vi "serial_02.vi"(0 "VISA resource name":refnum<visa-resource-name>="COM5") -> ()   [LabVIEW 2010]
doc: "The Basic Serial Read and Write example performs a Serial Port Read, a Serial Port Write, or a combination of these actions. The user selects the actions (read or write) on the front panel. If both are selected, the VI will write the data first, read data, and then close the VISA session that is opened to the port. This VI will wait until the specified number of bytes is received at the port. Only the number of bytes specified will be read.\n\nINSTRUCTIONS:\n1) Select the serial resource and configuration parameters (baud rate, data bits, parity, stop bits, flow control).\n2) Select the operations to be performed. \n3) Connect the serial port to your device. If no device is available, perform a loopback test by doing one of the following. Short pins 2 and 3 on a RS-232 cable or short pin 4 to pin 8 and pin 5 to pin 9 on a RS-485/422 cable. \n4) Run the VI to see the data read. (The \"read string\" will match the \"string to write\" if a loopback test was performed.)\n\nNote: The parameters set for the serial port must match the parameters of the connected instrument or device. In this example, the bytes to read parameter specifies the number of bytes that the serial port reads. If there were more bytes at the port than the number specified in bytes to read, those bytes would not be read. Also, if you specify to read more bytes than the number of bytes actually read, you might receive a timeout error message.\n\nOn the block diagram, the Configure Serial Port VI sets the configuration parameters. The front panel displays the controls used to configure the basic parameters, such as baud rate, data bits, and parity. Constants configure the other parameters the user probably does not need set. After the VISA Configure Serial Port VI opens the VISA session and configures the port, the VI passes the VISA resource name to other VIs that perform operations on that VISA resource. The VISA Write function sends a command to the serial device and the VISA Read function returns data based on the command. The VISA Close function then closes the reference to the serial device. It is important to close the reference; otherwise communication through with that port through protocols other than VISA might not be possible."
panel:
  in  "Start":bool=TRUE
  out "Meter":dbl(knob)=668.0 scale=0.0..1024.0
  out "Waveform Chart":i32(graph)=668
  # "Stop"
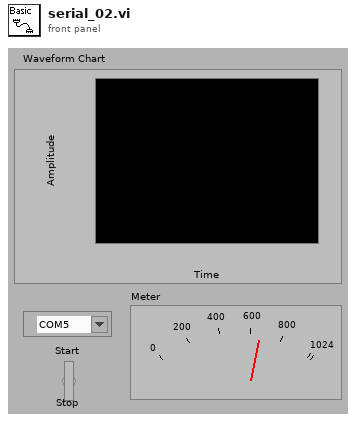
[diagram p1: front panel]
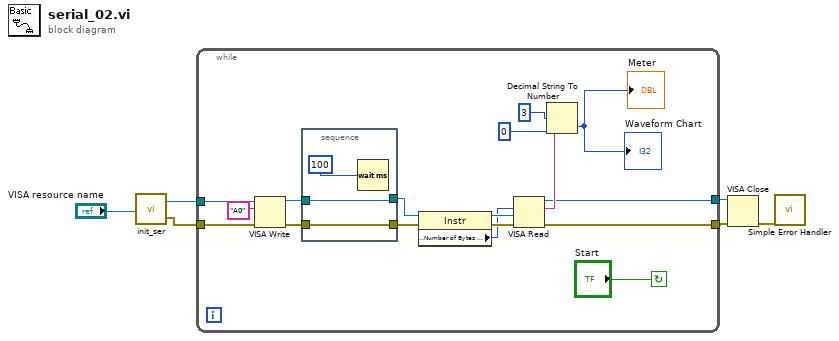
[diagram p0: block diagram]
diagram:
  n1 = call "init_ser.vi"("VISA resource name"="VISA resource name") -> ("VISA resource name out"=w4:refnum<visa-resource-name>, "error out"=w5:errorcluster)
  n2 = while {
    tunnel: w5 -> [w20]
    tunnel: w4 -> [w21]
    tunnel: [w9] -> w3
    tunnel: [w10] -> w2
    stop <- "Start" continue-if-true
    n3 = VISA Write(VISA resource name=w21, write buffer="A0" ("string to write"), error in (no error)=w20) -> (VISA resource name out=w19:refnum<visa-resource-name>, error out=w18:errorcluster)  [unwired: 1 out]
    n4 = stacked-sequence {
      tunnel: w19 -> [w25]
      tunnel: w18 -> [w24]
      tunnel: [w25] -> w8
      tunnel: [w24] -> w7
      frame #0 {
        n5 = Wait (ms)(milliseconds to wait=u32 100 ("delay before read (ms)")) -> ()  [unwired: 1 out]
      }
    }
    n6 = property class="Instr"(reference=w8, error in=w7) -> (reference out=w17:refnum<visa-resource-name>, error out=w16:errorcluster, "Serial Settings:Number of Bytes at Serial Port"=w15:u32)
    n7 = VISA Read(VISA resource name=w17, byte count=w15, error in (no error)=w16) -> (VISA resource name out=w10:refnum<visa-resource-name>, read buffer=w14:string, error out=w9:errorcluster)  [unwired: 1 out]
    n8 = Decimal String To Number(string=w14, offset=3, default (0L)=0) -> (number=→"Waveform Chart" →"Meter":i32)  [unwired: 1 out]
  }
  n9 = VISA Close(VISA resource name=w2, error in (no error)=w3) -> (error out=w1:errorcluster)
  n10 = call <vilib>:"Simple Error Handler.vi"("error in (no error)"=w1) -> ()  [unwired: 1 in, 8 out]
